vi "WPI_CANJaguar_ConfigMessagesCache.vi"(8 "Check All":bool, 9 "Config Message":T5={"Message ID"=0, "Needs Check"=TRUE, "Data"=[], "Mode"=FALSE}, 10 "Update":bool, 11 "CAN Jaguar Ref":T1={"DeviceStatus"={"status"=FALSE, "code"=0, "source"=""}, "Type"=enum."PWM", "PWM"={"PWM Channel"=enum."PWM 1", "DeadBand"={"Name"="", "maxPositivePwm"=0, "minPositivePwm"=0, "centerPwm"=0, "maxNegativePwm"=0, "minNegativePwm"=0, "angularRange"=0}}, "CAN"={"Device Number"=0, "SetOutput VI Ref"=variant(enum8{"Percent VBus", "Current", "Speed", "Position", "Voltage"} enum."Percent VBus"), "GetOutput VI Ref"=variant(refnum<k1> refnum), "Enable VI Ref"=variant(dbl 12.0), "Disable VI Ref"=variant(enum8{"Percent VBus", "Speed", "Position", "Slave", "Unchanged / Invalid", "Voltage Compensation", "Current", "Motion Profile"} enum."Percent VBus"), "Data"=variant}, "Invert"=FALSE}) -> (3 "Config Message Cache":T5[](array[typedef]))   [LabVIEW 2016]
uses:
  <vilib>/Rock Robotics/WPI/ThirdParty/CanMotor/CAN Jaguar/SubVIs/WPI_CANJaguar_ConfigMessage.ctl
  <vilib>/Rock Robotics/WPI/MotorControl/WPI_MotorControlDeviceRef.ctl
  <vilib>/Rock Robotics/WPI/MotorControl/WPI_MotorControlType.ctl
  <vilib>/Rock Robotics/SystemInterfaces/DIO/FPGA_DIOPWMChannel.ctl
  <vilib>/Rock Robotics/WPI/PWM/WPI_PWMDeadband.ctl
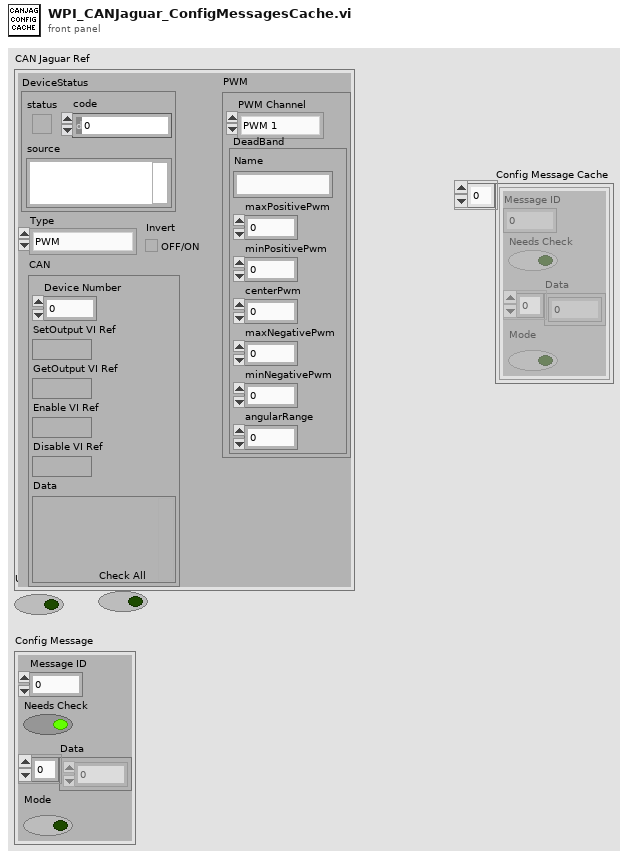
[diagram p1: front panel]
types:
  T1 = typedef "WPI_MotorControlDeviceRef.ctl" = cluster{"DeviceStatus":errorcluster, "Type":T2, "PWM":cluster{"PWM Channel":T3, "DeadBand":T4}, "CAN":cluster{"Device Number":u8, "SetOutput VI Ref":variant, "GetOutput VI Ref":variant, "Enable VI Ref":variant, "Disable VI Ref":variant, "Data":variant}, "Invert":bool}
  T2 = typedef "WPI_MotorControlType.ctl" = enum16{"PWM", "CAN"}
  T3 = typedef "FPGA_DIOPWMChannel.ctl" = enum8{"PWM 0", "PWM 1", "PWM 2", "PWM 3", "PWM 4", "PWM 5", "PWM 6", "PWM 7", "PWM 8", "PWM 9", "PWM MXP 0", "PWM MXP 1", "PWM MXP 2", "PWM MXP 3", "PWM MXP 4", "PWM MXP 5", "PWM MXP 6", "PWM MXP 7", "PWM MXP 8", "PWM MXP 9", "Invalid"}
  T4 = typedef "WPI_PWMDeadband.ctl" = cluster{"Name":string, "maxPositivePwm":i32, "minPositivePwm":i32, "centerPwm":i32, "maxNegativePwm":i32, "minNegativePwm":i32, "angularRange":u16}
  T5 = typedef "WPI_CANJaguar_ConfigMessage.ctl" = cluster{"Message ID":u32, "Needs Check":bool, "Data":u8[], "Mode":bool}
  T6 = cluster{"Device Number":u8, "Config Messages":T5[]}[]
  T7 = cluster{"Device Number":u8, "Config Messages":T5[]}
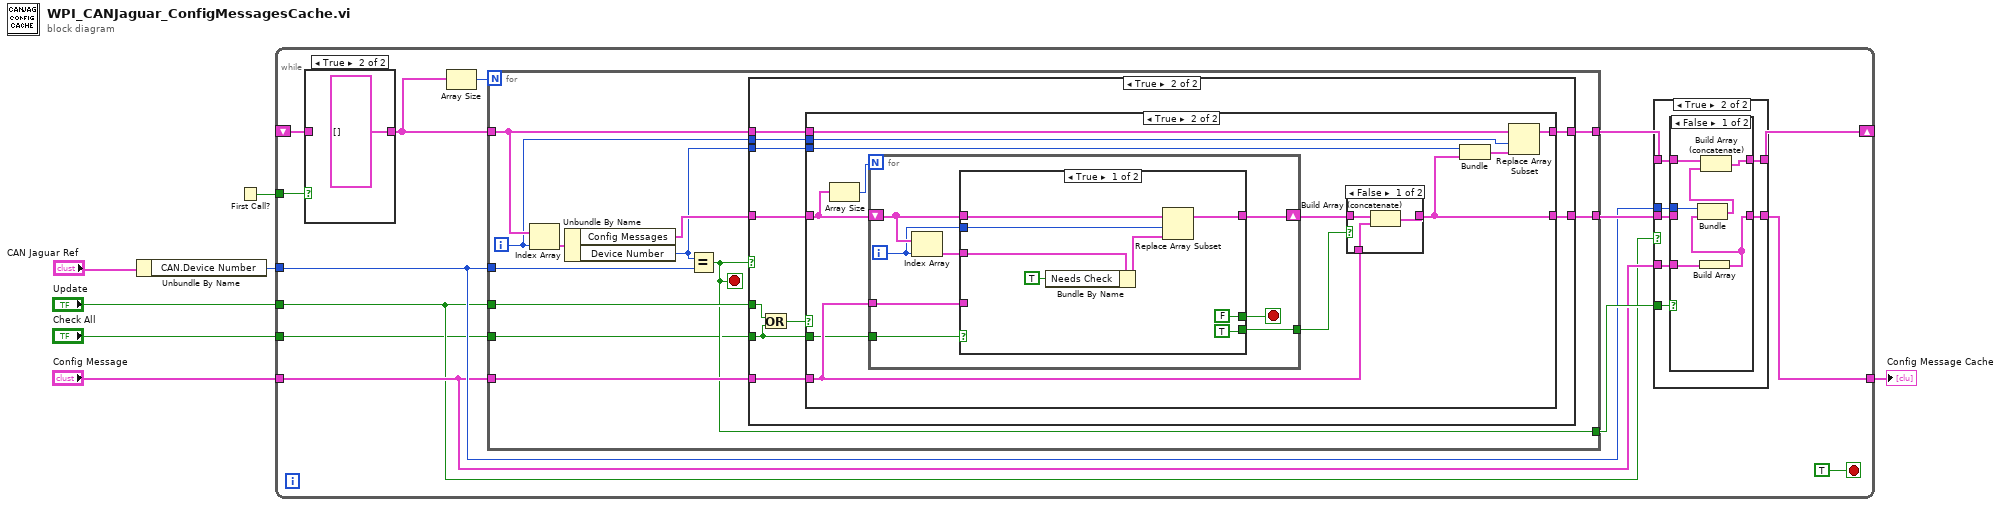
[diagram p0: block diagram]
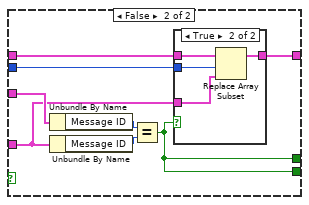
[diagram p7: hidden frame]
diagram:
  n1 = Unbundle By Name("CAN Jaguar Ref") -> ("CAN.Device Number"=w3:u8)
  n2 = First Call?() -> (First Call?: T/F=w2:bool)
  n3 = while {
    tunnel: "Config Message" -> [w10]
    tunnel: "Update" -> [w9]
    tunnel: w2 -> [w20]
    tunnel: [w13] -> w5
    shift-right: [w15] -> _
    shift-left: _ -> [w19]
    tunnel: w3 -> [w11]
    tunnel: "Check All" -> [w8]
    stop <- TRUE stop-if-true
    n4 = case shown="True" w20 {
      tunnel: [w109 T6 []] -> w17
      tunnel: w19 -> [w109 _]
      frame False {
      }
      frame True {
      }
    }
    n5 = Array Size(array=w17) -> (size(s)=w18:i32)
    n6 = for {
      N: w18 -> [_]
      tunnel: w9 -> [w50]
      tunnel: w10 -> [w49]
      tunnel: w11 -> [w46]
      tunnel: [w45] -> w16
      tunnel: [w40] -> w12
      tunnel: w17 -> [w44]
      tunnel: [w48] -> w14
      tunnel: w8 -> [w39]
      i -> [w41]
      stop <- w45 stop-if-true
      n7 = Index Array(array=w44, index=w41) -> (element=w47:T7)
      n8 = Unbundle By Name(w47) -> ("Config Messages"=w43:T5[], "Device Number"=w42:u8)
      n9 = Equal?(x=w42, y=w46) -> (x = y?=w45:bool)
      n10 = case shown="True" w45 {
        tunnel: w50 -> [_ w53]
        tunnel: w49 -> [_ w61]
        tunnel: [w51 w59] -> w48
        tunnel: w43 -> [_ w60]
        tunnel: w44 -> [w51 w58]
        tunnel: w42 -> [_ w57]
        tunnel: w41 -> [_ w56]
        tunnel: [_ w55] -> w40
        tunnel: w39 -> [_ w54]
        frame False {
        }
        frame True {
          n11 = Or(x=w53, y=w54) -> (x .or. y?=w52:bool)
          n12 = case shown="True" w52 {
            tunnel: w61 -> [_ w71]
            tunnel: [w63 w68] -> w55
            tunnel: w60 -> [w63 w73]
            tunnel: [w62 w69] -> w59
            tunnel: w58 -> [w62 w70]
            tunnel: w57 -> [_ w67]
            tunnel: w56 -> [_ w65]
            tunnel: w54 -> [_ w64]
            frame False {
            }
            frame True {
              n13 = Array Size(array=w73) -> (size(s)=w74:i32)
              n14 = for {
                N: w74 -> [_]
                tunnel: w71 -> [w82]
                tunnel: [w81] -> w75
                tunnel: w64 -> [w80]
                shift-right: [w84] -> w72
                shift-left: w73 -> [w85]
                i -> [w83]
                stop <- w87 stop-if-true
                n15 = Index Array(array=w85, index=w83) -> (element=w86:T5)
                n16 = case shown="True" w80 {
                  tunnel: [FALSE w96] -> w87
                  tunnel: w86 -> [w90 w101]
                  tunnel: w85 -> [w95 w100]
                  tunnel: [w94 w99] -> w84
                  tunnel: w83 -> [w93 w98]
                  tunnel: w82 -> [_ w97]
                  tunnel: [TRUE w96] -> w81
                  frame True {
                    n17 = Bundle By Name(cluster=w90, "Needs Check"=TRUE) -> (w89:T5)
                    n18 = Replace Array Subset(array=w95, new element=w89, index=w93) -> (w94:T5[])
                  }
                  frame False {
                    n19 = Unbundle By Name(w101) -> ("Message ID"=w103:u32)
                    n20 = Unbundle By Name(w97) -> ("Message ID"=w102:u32)
                    n21 = Equal?(x=w103, y=w102) -> (x = y?=w96:bool)
                    n22 = case shown="True" w96 {
                      tunnel: w100 -> [w104 w108]
                      tunnel: [w104 w107] -> w99
                      tunnel: w98 -> [_ w106]
                      tunnel: w97 -> [_ w105]
                      frame False {
                      }
                      frame True {
                        n23 = Replace Array Subset(array=w108, new element=w105, index=w106) -> (w107:T5[])
                      }
                    }
                  }
                }
              }
              n24 = case shown="False" w75 {
                tunnel: [w77 w79] -> w68
                tunnel: w72 -> [w78 w79]
                tunnel: w71 -> [w76 _]
                frame False {
                  n25 = Build Array (concatenate)(w78, w76) -> (w77:T5[])
                }
                frame True {
                }
              }
              n26 = Bundle("Device Number"=w67, "Config Messages"=w68) -> (w66:T7)  [unwired: 1 in]
              n27 = Replace Array Subset(array=w70, new element=w66, index=w65) -> (w69:T6)
            }
          }
        }
      }
    }
    n28 = case shown="True" w9 {
      tunnel: w16 -> [_ w30]
      tunnel: [w23 w29] -> w15
      tunnel: w14 -> [w23 w28]
      tunnel: [w22 w27] -> w13
      tunnel: w12 -> [w22 w26]
      tunnel: w11 -> [_ w25]
      tunnel: w10 -> [_ w24]
      frame False {
      }
      frame True {
        n29 = case shown="False" w30 {
          tunnel: [w33 w38] -> w29
          tunnel: w28 -> [w35 w38]
          tunnel: [w31 w37] -> w27
          tunnel: w26 -> [_ w37]
          tunnel: w25 -> [w36 _]
          tunnel: w24 -> [w32 _]
          frame False {
            n30 = Build Array(w32) -> (w31:T5[])
            n31 = Bundle("Device Number"=w36, w31) -> (w34:cluster{"Device Number":u8, T5[]})  [unwired: 1 in]
            n32 = Build Array (concatenate)(w35, w34) -> (w33:T6)
          }
          frame True {
          }
        }
      }
    }
  }
  "Config Message Cache" <- w5
